vi "AMC e.bloxx Get Device Information.vi"(8 "error in (no error)":errorcluster, 10 "Module Address":i32, 11 "VISA Resource Name":refnum<visa-resource-name>) -> (0 "error out":errorcluster, 1 "Channel Count":i32, 2 "Location":string, 3 "VISA Resource Name out":refnum<visa-resource-name>, 5 "Serial Number":i32)   [LabVIEW 2013]
doc: "<B>AMC - Analytik & Messtechnik GmbH Chemnitz</B>\n\nLabVIEW Drivers for e.bloxx series from Gantner Instruments\n\nThis VI reads the device information from the module specified by <B>Module Address</B>."
uses:
  <vilib>/Utility/error.llb/whitespace.ctl
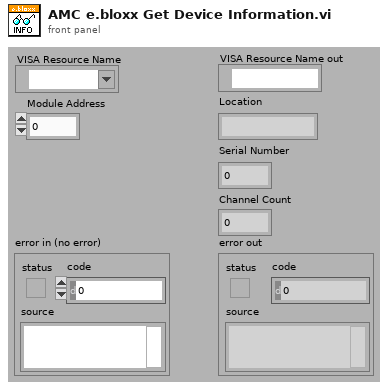
[diagram p1: front panel]
types:
  T1 = typedef "whitespace.ctl" = u16
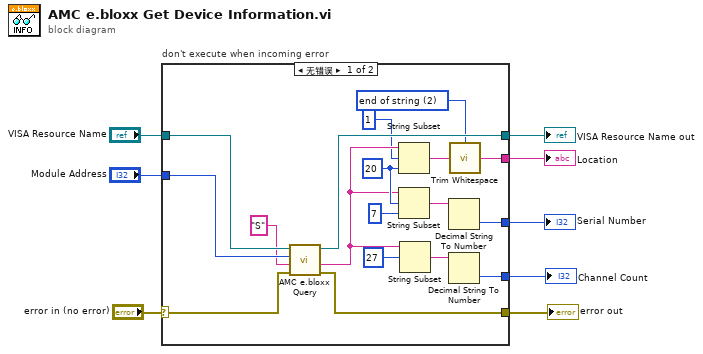
[diagram p0: block diagram]
diagram:
  n1 = case "don't execute when incoming error" shown="无错误" "error in (no error)" {
    selector: "error in (no error)" -> [w26 w28]
    tunnel: [w22 w28] -> w7
    tunnel: "VISA Resource Name" -> [w24 w27]
    tunnel: "Module Address" -> [w25 _]
    tunnel: [w21 w27] -> w4
    tunnel: [w12 _] -> w3
    tunnel: [w10 _] -> w2
    tunnel: [w9 _] -> w1
    frame No Error {
      w11 = T1 2 items=["both", "start of string", "end of string"] ("location (both)")
      w20 = 20 ("length (rest)")
      n2 = call "AMC e.bloxx Query.vi"("error in (no error)"=w26, "Module Command"="S", "Module Address"=w25, "VISA Resource Name"=w24) -> ("error out"=w22:errorcluster, "Module Response"=w16:string, "VISA Resource Name out"=w21:refnum<visa-resource-name>)  [unwired: 5 in]
      n3 = String Subset(string=w16, offset (0)=1, length (rest)=w20) -> (substring=w13:string)
      n4 = String Subset(string=w16, offset (0)=w20, length (rest)=7 ("length (rest)")) -> (substring=w19:string)
      n5 = String Subset(string=w16, offset (0)=27) -> (substring=w15:string)  [unwired: 1 in]
      n6 = Decimal String To Number(string=w19) -> (number=w10:i32)  [unwired: 2 in, 1 out]
      n7 = Decimal String To Number(string=w15) -> (number=w9:i32)  [unwired: 2 in, 1 out]
      n8 = call <vilib>:"Trim Whitespace.vi"("string"=w13, "location (both)"=w11) -> ("trimmed string"=w12:string)
    }
    frame Error {
    }
  }
  "error out" <- w7
  "VISA Resource Name out" <- w4
  "Location" <- w3
  "Serial Number" <- w2
  "Channel Count" <- w1
